vi "DisableInMemory.vi"(0 "reference in":refnum<class "G#RemoteProxy.lvclass">, 5 "error in (no error)":errorcluster) -> (14 "reference out":refnum<class "G#RemoteProxy.lvclass">, 19 "error out":errorcluster)   [LabVIEW 2017, in "G#RemoteProxy.lvclass"]
doc: "Disables the in memory flag. It seems like there is a an aggregated object that is not in the project."
uses:
  <vilib>/addons/_AddQ/G#Debugger/G#RemoteProxy/G#RemoteProxy.lvclass
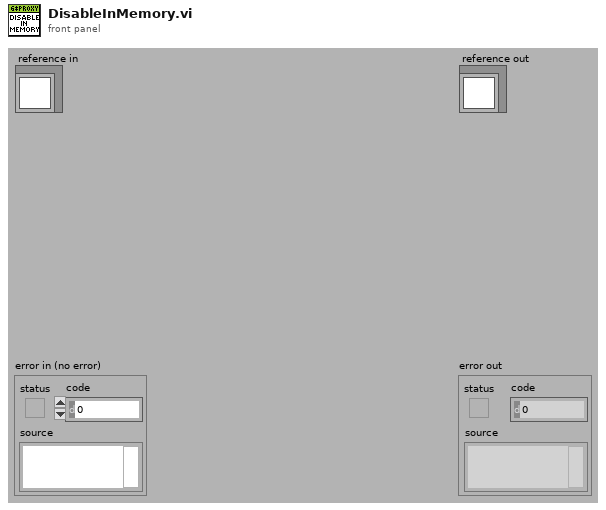
[diagram p1: front panel]
types:
  T1 = typedef "G#RemoteProxy.lvclass/ObjectAttributesRef.ctl" = refnum<data-value>
  T2 = typedef "G#RemoteProxy.lvclass/ObjectAttributesProxy.ctl" = cluster{"class hierarchy":T3[], "class name":string, "lvlib hierarchy":string[], "full class name":string, "id":u32, "owner":string, "RemoteRef":refnum<class "G#Object.lvclass">, "object name":string, "attributes":variant[], "connection ID":refnum<k5>, "address":u32, "occurrence":refnum<k4>, "ProxyClassRef":refnum<class "G#RemoteProxy.lvclass">, "InMemory?":bool, "ToString":string}
  T3 = typedef "G#Object.lvclass/G#Object_ClassHierarchy.ctl" = cluster{"ClassName":string, "FullClassName":string, "ClassPath":path, "IsLeaf":bool}
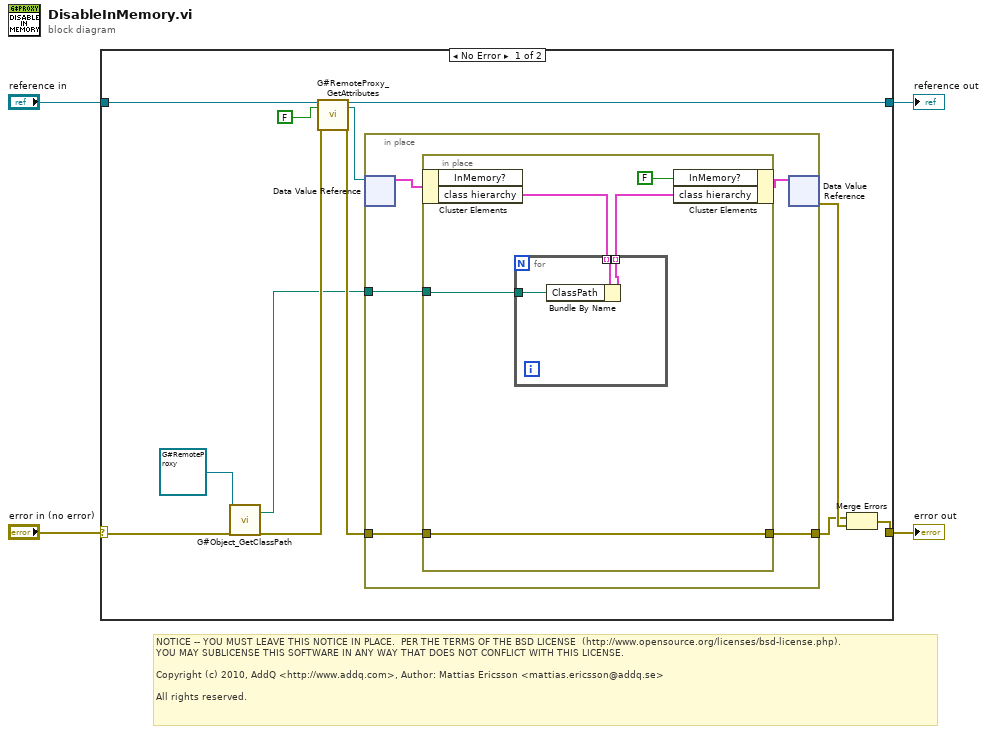
[diagram p0: block diagram]
diagram:
  # "NOTICE -- YOU MUST LEAVE THIS NOTICE IN PLACE.  PER THE TERMS OF THE BSD LICENSE  (http://www.opensource.org/licenses/bsd-license.php).\nYOU MAY SUBLICENSE THIS SOFTWARE IN ANY WAY THAT DOES NOT CONFLICT WITH THIS LICENSE.\n\nCopyright (c) 2010, AddQ <http://www.addq.com>, Author: Mattias Ericsson <mattias.ericsson@addq.se>\n\nAll rights reserved."
  n1 = case shown="No Error" "error in (no error)" {
    selector: "error in (no error)" -> [w7 w31]
    tunnel: [w16 w31] -> w3
    tunnel: [w10 w30] -> w1
    tunnel: "reference in" -> [w13 w30]
    frame No Error {
      n2 = call-dynamic "G#Object_GetClassPath.vi"("reference in"=refnum<class "G#RemoteProxy.lvclass"> refnum ("G#RemoteProxy.lvclass"), "error in (no error)"=w7) -> ("class path"=w5:path, "error out"=w6:errorcluster)  [unwired: 15 in, 1 out]
      n3 = call <vilib>:"G#RemoteProxy_GetAttributes.vi"("reference in"=w13, "return data? (T)"=FALSE, "error in (no error)"=w6) -> ("reference out"=w10:refnum<class "G#RemoteProxy.lvclass">, "attributes ref"=w9:T1, "error out"=w11:errorcluster)  [unwired: 13 in, 1 out]
      n4 = in-place {
        in-place-border: w11 -> [w19]
        in-place-border: [w17] -> w14
        in-place-border: w5 -> [w18]
        n5 = in-place-dvr #1(w9) -> (w20:T2)  [unwired: 1 out]
        n6 = in-place {
          in-place-border: w19 -> [w22]
          in-place-border: w18 -> [w23]
          in-place-border: [w22] -> w17
          n7 = in-place-cluster #2(w20) -> ("class hierarchy"=w25:T3[])  [unwired: 1 out]
          n8 = for {
            tunnel: w25 -> [w29] mode=indexing
            tunnel: [w28] -> w24 mode=indexing
            tunnel: w23 -> [w27]
            n9 = Bundle By Name(cluster=w29, "ClassPath"=w27) -> (w28:T3)
          }
          n10 = in-place-cluster #2("InMemory?"=FALSE, "class hierarchy"=w24) -> (w21:T2)
        }
        n11 = in-place-dvr #1(w21) -> (w15:errorcluster)  [unwired: 1 out]
      }
      n12 = Merge Errors(w14, w15) -> (w16:errorcluster)
    }
    frame Error {
    }
  }
  "error out" <- w3
  "reference out" <- w1
